vi "Read from stderr.vi"(11 "subprocess in":refnum<class "Buffered Subprocess.lvclass">) -> (2 "data":u8[](array[numeric]), 3 "subprocess out":refnum<class "Buffered Subprocess.lvclass">)   [LabVIEW 2020, in "NI_Subprocess.lvlib" / "Buffered Subprocess.lvclass"]
uses:
  <vilib>/Subprocess/Buffered Subprocess/Buffered Subprocess.lvclass
  <vilib>/Subprocess/Buffered Subprocess/Buffered Subprocess.lvclass/Buffered Subprocess.ctl
  <vilib>/Array/Bytestream/Bytestream.lvclass/Bytestream.ctl
  <vilib>/Array/Bytestream/Bytestream.lvclass
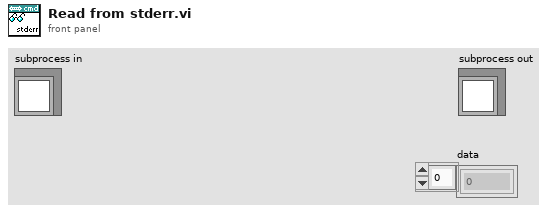
[diagram p1: front panel]
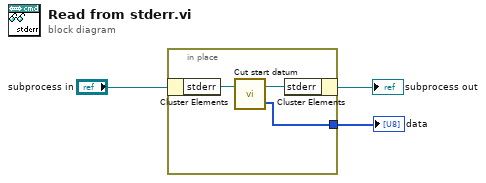
[diagram p0: block diagram]
diagram:
  n1 = in-place {
    in-place-border: [w4] -> w1
    n2 = in-place-cluster #1("subprocess in") -> ("stderr"=w6:refnum<class "Bytestream.lvclass">)
    n3 = call <vilib>:"Cut start datum.vi"("bytestream"=w6) -> ("data"=w4:u8[], "bytestream out"=w5:refnum<class "Bytestream.lvclass">)  [unwired: 1 in]
    n4 = in-place-cluster #1("stderr"=w5) -> (→"subprocess out":refnum<class "Buffered Subprocess.lvclass">)
  }
  "data" <- w1
